vi "Simple Digital Input.vi"() -> ()   [LabVIEW 2013]
doc: "This example shows how to read values from a digital channel.\n\nIt will display the digital value as Low (LED off) or High (LED on).\n\nThis example works with the NI 9403 module connected to a Digital Sidecar. The Digital Sidecar should have 12V applied to the WAGO connector. Note that the digital channels are pulled high when floating. This means that if you want to read a limit switch, you would need to connect one end of the switch to SIG and the other end to (-). The the LED would be On when the switch is open and Off when the switch is closed."
uses:
  <vilib>/Rock Robotics/SystemInterfaces/DIO/FPGA_DIOChannel.ctl
  <vilib>/Rock Robotics/SystemInterfaces/Typedef/FPGA_TypedefDigitalModule.ctl
panel:
  in  "DIO Module":T1
  out "Digital Input Value":bool
  in  "DIO Channel":T2
  in  "stop":bool
  # "Wiring Diagram for Digital Sidecar connected to an NI 9403"
  # "Set these inputs before running."
  # "PWR"
  # "SIG"
  # "(-)"
  # "14\n13\n12\n11\n10\n9\n8\n7\n6\n5\n4\n3\n2\n1"
  # "DIGITAL I/O"
  # "TTL Signal"
  # "This shows wiring for a TTL signal.  To read a switch, wire one side of the switch to SIG and the other side to (-).  The LED will be On when the switch is open and Off when the switch is closed."
  # "Digital Sidecar"
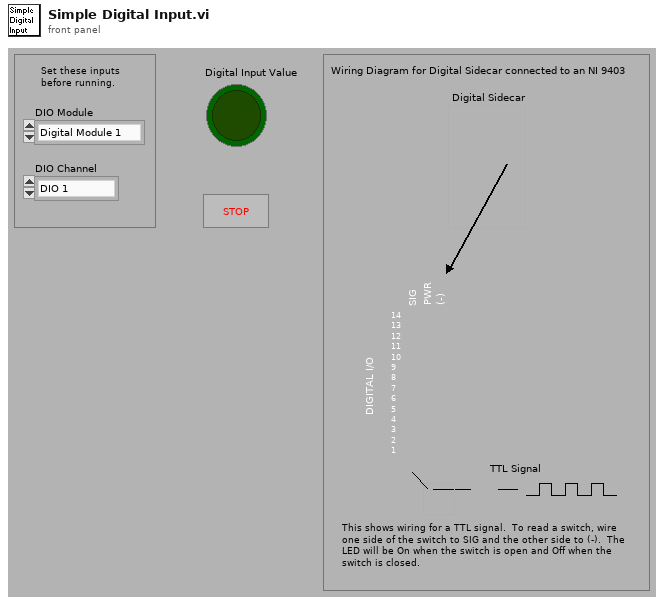
[diagram p1: front panel]
types:
  T1 = typedef "FPGA_TypedefDigitalModule.ctl" = enum16{"Digital Module 1", "Digital Module 2"}
  T2 = typedef "FPGA_DIOChannel.ctl" = enum8{"DIO 1", "DIO 2", "DIO 3", "DIO 4", "DIO 5", "DIO 6", "DIO 7", "DIO 8", "DIO 9", "DIO 10", "DIO 11", "DIO 12", "DIO 13", "DIO 14", "Invalid"}
  T3 = typedef "WPI_DigitalInputDevRef.ctl" = cluster{"DevStatus":errorcluster, "DIO Channel":T2, "Digital Module":T1}
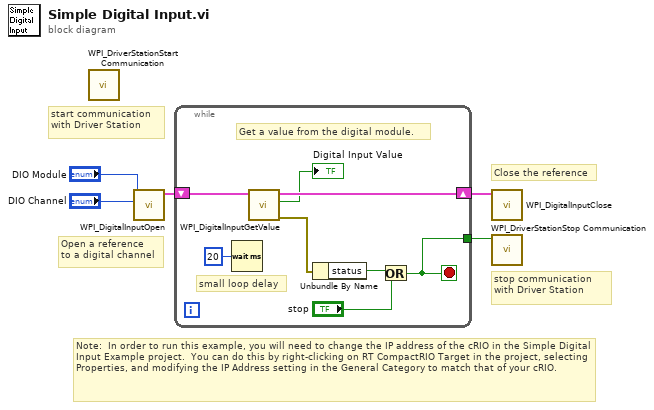
[diagram p0: block diagram]
diagram:
  # "stop communication with Driver Station"
  # "start communication with Driver Station"
  # "Note:  In order to run this example, you will need to change the IP address of the cRIO in the Simple Digital Input Example project.  You can do this by right-clicking on RT CompactRIO Target in the project, selecting Properties, and modifying the IP Address setting in the General Category to match that of your cRIO."
  # "Close the reference"
  # "Open a reference\nto a digital channel"
  n1 = call <vilib>:"WPI_DriverStationStart Communication.vi"() -> ()  [unwired: 1 in, 11 out]
  n2 = call <vilib>:"WPI_DigitalInputOpen.vi"("DIO Channel"="DIO Channel", "Digital Module (Module 1)"="DIO Module") -> ("DigitalInputDevRef"=w4:T3)  [unwired: 1 in, 8 out]
  n3 = while {
    shift-right: [w12] -> w3
    shift-left: w4 -> [w13]
    tunnel: [w8] -> w2
    stop <- w8 stop-if-true
    # "small loop delay"
    # "Get a value from the digital module."
    n4 = Wait (ms)(milliseconds to wait=u32 20) -> ()  [unwired: 1 out]
    n5 = call <vilib>:"WPI_DigitalInputGetValue.vi"("DigitalInputDevRef"=w13) -> ("error out"=w7:errorcluster, "Value"=→"Digital Input Value":bool, "DigitalInputDevRef"=w12:T3)  [unwired: 1 in, 7 out]
    n6 = Unbundle By Name(w7) -> ("status"=w9:bool)
    n7 = Or(x=w9, y="stop") -> (x .or. y?=w8:bool)
  }
  n8 = call <vilib>:"WPI_DigitalInputClose.vi"("DigitalInputDevRef"=w3) -> ()  [unwired: 1 in, 10 out]
  n9 = call <vilib>:"WPI_DriverStationStop Communication.vi"("StopCommunication"=w2) -> ()  [unwired: 1 in, 10 out]
